vi "数据查询_仪器数据.vi"() -> ()   [LabVIEW 2016, in "数据查询.lvlib"]
uses:
  <vilib>/Utility/miscctls.llb/LVPointTypeDef.ctl
  <vilib>/Utility/miscctls.llb/LVRowAndColumnUnsignedTypeDef.ctl
  <userlib>/_OpenG.lib/array/array.llb/Sort 2D Array (String)__ogtk.vi
  <vilib>/ptbypt/NI_PtbyPt.lvlib
panel:
  in  "显示关键参数":bool
  in  "剔除异常数据":bool
  in  "数据类型":string(combo)="全部数据"
  in  "列表框":i32(listbox)
  in  "页":i32 format="第%.0f页"
  in  "每页条数":i32=1000
  in  "向后按钮":bool
  in  "向前按钮":bool
  in  "导出":bool
  in  "测量模式":string(combo)="全部数据"
  in  "查询":bool
  in  "结束日期":string="2050/01/01"
  in  "起始日期":string="2010/01/01"
  out "数据表":string[][](table)
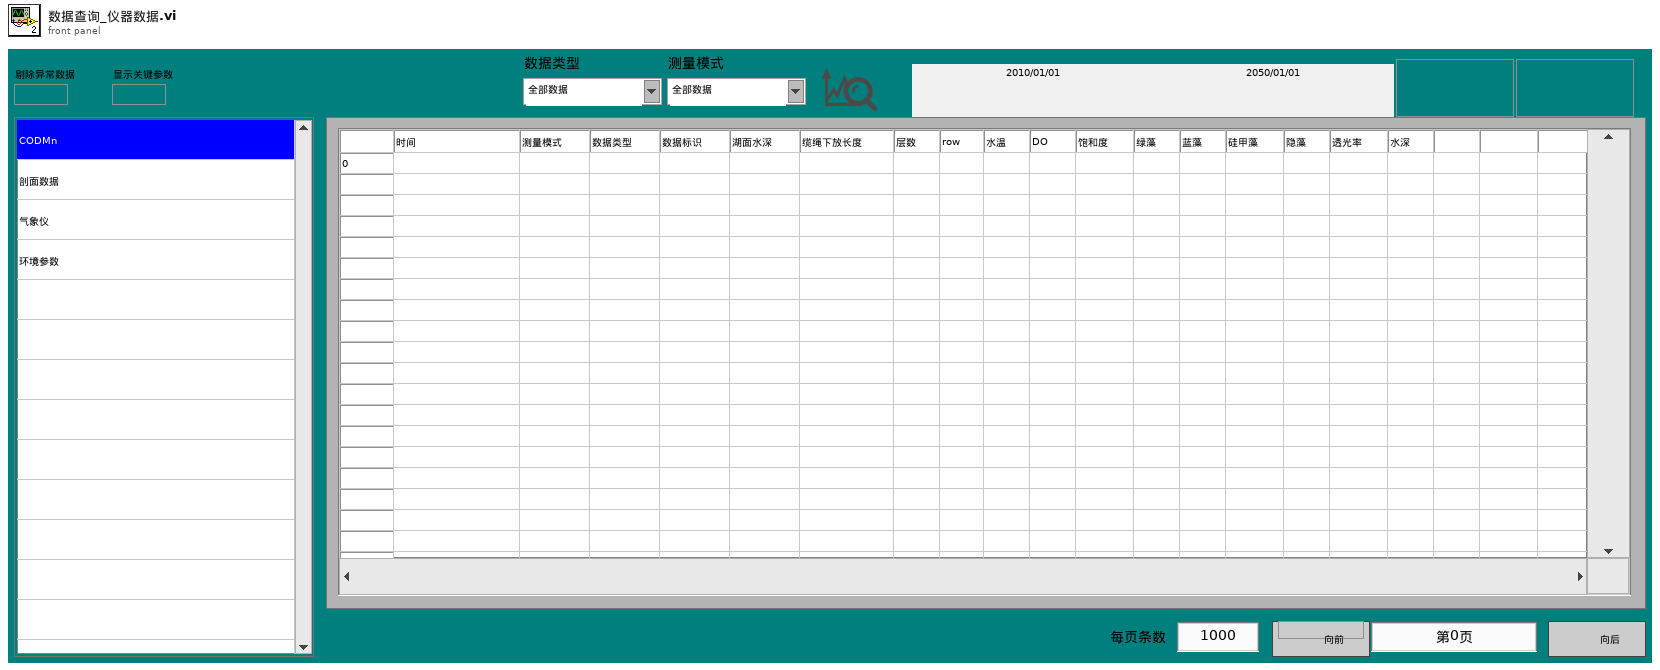
[diagram p1: front panel]
types:
  T1 = typedef "LVPointTypeDef.ctl" = cluster{"Horizontal":i16, "Vertical":i16}
  T2 = typedef "LVDateTimeRec.ctl" = cluster{"秒数的小数部分":dbl, "秒":i32, "分":i32, "时":i32, "日":i32, "月":i32, "年":i32, "天数（周）":i32, "天数（年）":i32, "DST":i32}
  T3 = typedef "数据查询菜单.xctl/数据 1.ctl" = enum32{"数据查询", "仪器数据", "仪器日志", "报警信息", "校准日志"}
  T4 = enum8{"Enabled", "Disabled", "Disabled and Grayed Out"}
  T5 = typedef "LVRowAndColumnUnsignedTypeDef.ctl" = cluster{"Row":u32, "Column":u32}
  T6 = typedef "数据库类型.ctl" = enum16{"Access", "SQLite"}
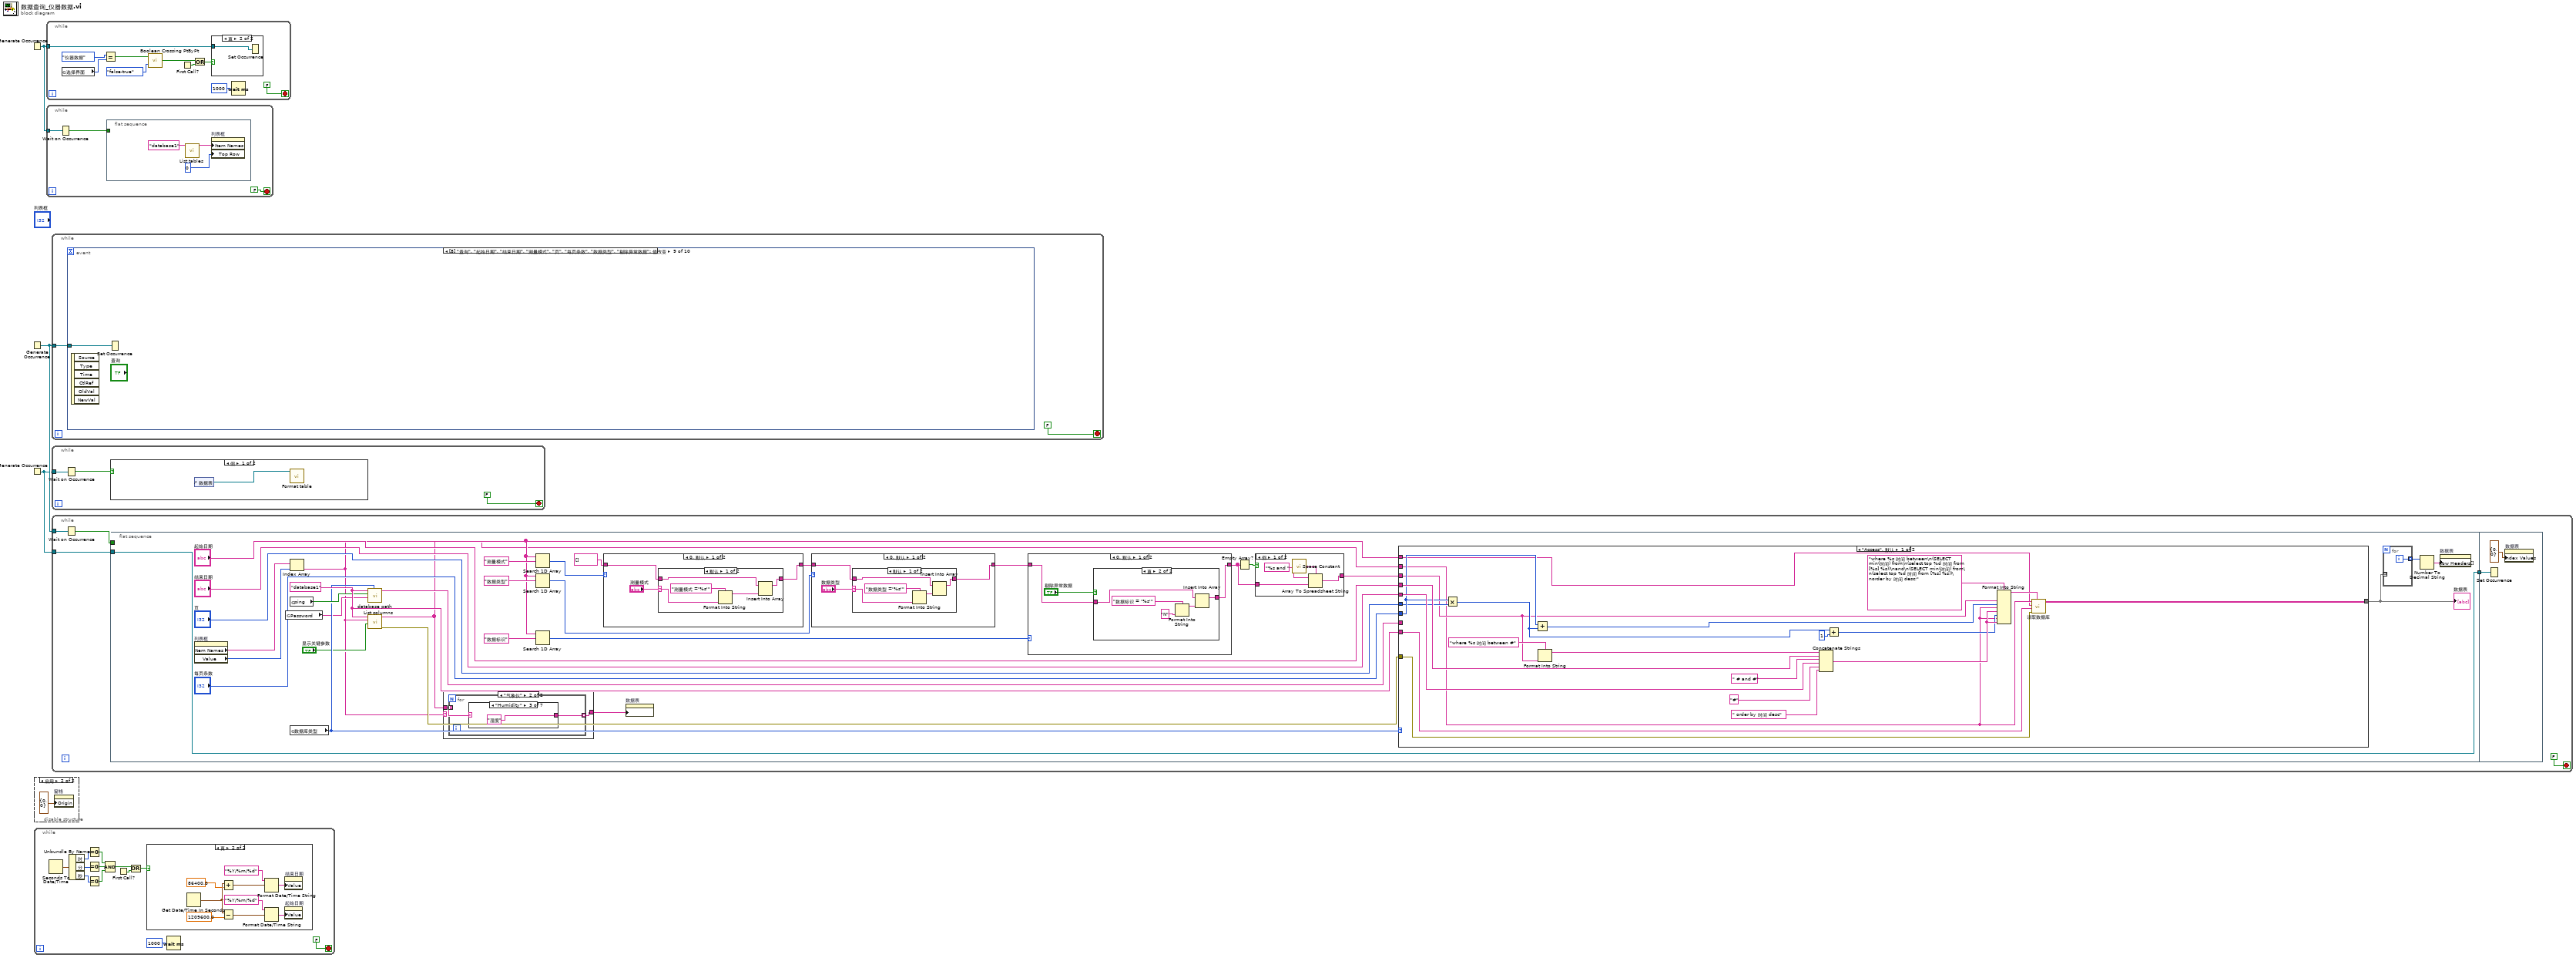
[diagram p0: block diagram]
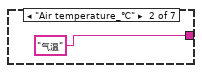
[diagram p6: hidden frame]
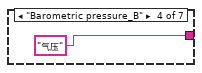
[diagram p7: hidden frame]
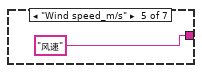
[diagram p8: hidden frame]
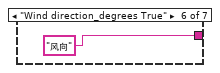
[diagram p9: hidden frame]
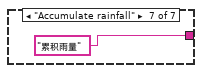
[diagram p10: hidden frame]
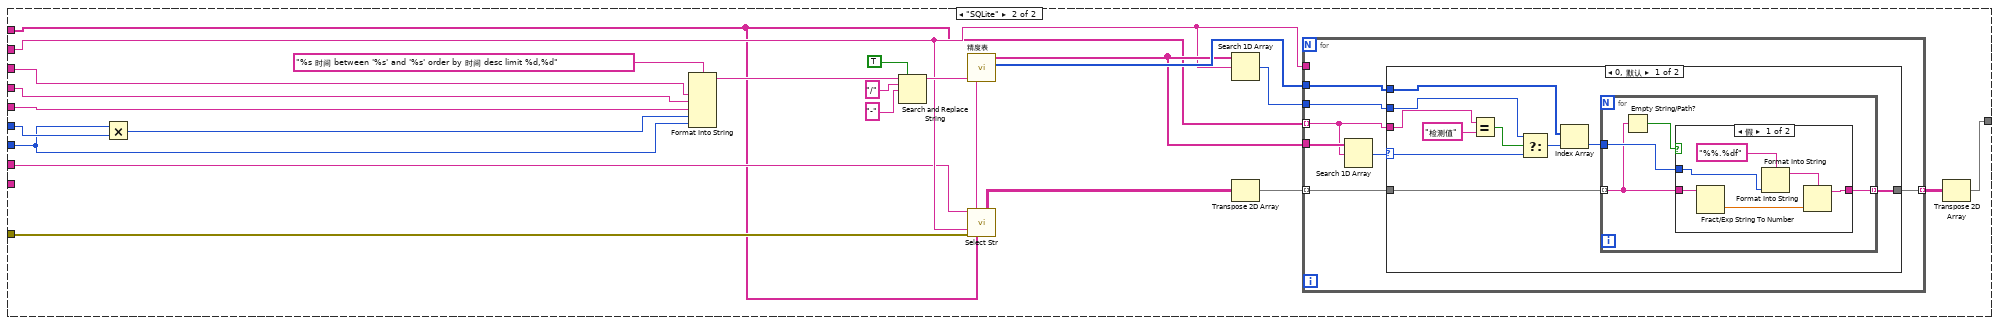
[diagram p11: hidden frame]
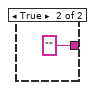
[diagram p14: hidden frame]
diagram:
  n1 = Generate Occurrence() -> (w1:refnum<k4>)
  n2 = Generate Occurrence() -> (w3:refnum<k4>)
  n3 = Generate Occurrence() -> (w2:refnum<k4>)
  n4 = disable-structure shown="启用" {
    frame Disabled {
    }
    frame Enabled {
      n5 = property on="窗格" class="Pane"("Origin"=T1 {"Horizontal"=0, "Vertical"=0} ("原点")) -> ()  [unwired: 2 in, 2 out]
    }
  }
  n6 = while {
    stop <- FALSE stop-if-true
    n7 = Seconds To Date/Time() -> (date time rec=w16:T2)  [unwired: 2 in]
    n8 = Unbundle By Name(w16) -> ("时"=w15:i32, "分"=w14:i32, "秒"=w13:i32)
    n9 = Equal To 0?(x=w15) -> (x = 0?=w12:bool)
    n10 = Equal To 0?(x=w14) -> (x = 0?=w11:bool)
    n11 = Equal To 0?(x=w13) -> (x = 0?=w10:bool)
    n12 = Compound Arithmetic op=AND ("复合运算")(w12, w11, w10) -> (w7:bool)
    n13 = First Call?() -> (First Call?: T/F=w6:bool)
    n14 = Or(x=w7, y=w6) -> (x .or. y?=w5:bool)
    n15 = case shown="真" w5 {
      frame False {
      }
      frame True {
        n16 = Get Date/Time In Seconds() -> (seconds since 1Jan1904=w21:timestamp)
        n17 = Add(x=w21, y=86400.0) -> (x+y=w19:timestamp)
        n18 = Subtract(x=w21, y=1209600.0) -> (x-y=w22:timestamp)
        n19 = Format Date/Time String(time format string (%c)="%Y/%m/%d" ("时间格式字符串(%c)"), seconds (now)=w19) -> (date/time string=w18:string)  [unwired: 1 in]
        n20 = Format Date/Time String(time format string (%c)="%Y/%m/%d" ("时间格式字符串(%c)"), seconds (now)=w22) -> (date/time string=w24:string)  [unwired: 1 in]
        n21 = property on="结束日期" class="Str"("Value"=w18) -> ()  [unwired: 2 in, 2 out]
        n22 = property on="起始日期" class="Str"("Value"=w24) -> ()  [unwired: 2 in, 2 out]
      }
    }
    n23 = Wait (ms)(milliseconds to wait=u32 1000 ("等待时间（毫秒）")) -> ()  [unwired: 1 out]
  }
  n24 = while {
    tunnel: w1 -> [w33]
    stop <- FALSE stop-if-true
    n25 = global read "全局变量.vi" "选择界面"() -> (w32:T3)
    n26 = Equal?(x=数据_1."仪器数据", y=w32) -> (x = y?=w30:bool)
    n27 = call <vilib>:"Boolean Crossing PtByPt.vi"("direction"=enum16{"either", "false-true", "true-false"}."false-true", "input"=w30) -> ("crossing"=w28:bool)  [unwired: 1 in]
    n28 = First Call?() -> (First Call?: T/F=w26:bool)
    n29 = Or(x=w28, y=w26) -> (x .or. y?=w27:bool)
    n30 = case shown="真" w27 {
      tunnel: w33 -> [_ w36]
      frame False {
      }
      frame True {
        n31 = Set Occurrence(w36) -> ()
      }
    }
    n32 = Wait (ms)(milliseconds to wait=u32 1000 ("等待时间（毫秒）")) -> ()  [unwired: 1 out]
  }
  n33 = while {
    tunnel: w1 -> [w38]
    stop <- FALSE stop-if-true
    n34 = Wait on Occurrence(2:w38) -> (0:w37:bool)  [unwired: 2 in]
    n35 = flat-sequence {
      tunnel: w37 -> [_]
      frame #0 {
        n36 = call "List tables.vi"("database"="database1") -> ("tables"=w40:string[])  [unwired: 9 in, 1 out]
        n37 = property on="列表框" class="LstBox (严格)"("Item Names"=w40, "Top Row"=0 ("顶行")) -> ()  [unwired: 2 in, 2 out]
      }
    }
  }
  n38 = while {
    tunnel: w3 -> [w43]
    stop <- FALSE stop-if-true
    n39 = event shown="[8] \"查询\", \"起始日期\", \"结束日期\", \"测量模式\", \"页\", \"每页条数\", \"数据类型\", \"剔除异常数据\": 值改变" {
      selector: _ -> [_ _ _ _ _ _ _ _ _ _]
      dyn-events: _ -> [_ _ _ _ _ _ _ _ _ _]
      timeout: _ -> [_ _ _ _ _ _ _ _ _ _]
      tunnel: w43 -> [_ _ _ _ _ _ _ _ w110 w112]
      event Timeout {
        n40 = event-data() -> ()  [unwired: 1 in, 3 out]
      }
      event "查询": Mouse Down {
        n41 = event-data() -> ()  [unwired: 1 in, 8 out]
        n42 = property on="页" class="DigNum (严格)"("Value"=0 ("页")) -> ()  [unwired: 2 in, 2 out]
      }
      event "每页条数": Mouse Down {
        n43 = event-data() -> ("CtlRef"=w47:refnum<vi>)  [unwired: 1 in, 7 out]
        n44 = property on="页" class="DigNum (严格)"("Value"=0 ("页")) -> ()  [unwired: 2 in, 2 out]
        n45 = property class="DigNum (严格)"(reference=w47) -> (reference out=w48:refnum<vi>, "Value"=w50:i32)  [unwired: 1 in, 1 out]
        n46 = call "数字键盘.vi"("OldNumber"=w50) -> ("NewNumber"=w49:sgl)
        n47 = property class="DigNum (严格)"(reference=w48, "Val(Sgnl)"=w49) -> ()  [unwired: 1 in, 2 out]
      }
      event "页": Mouse Down {
        n48 = event-data() -> ("CtlRef"=w51:refnum<vi>)  [unwired: 1 in, 7 out]
        n49 = property class="DigNum (严格)"(reference=w51) -> (reference out=w52:refnum<vi>, "Value"=w54:i32)  [unwired: 1 in, 1 out]
        n50 = call "数字键盘.vi"("OldNumber"=w54) -> ("NewNumber"=w53:sgl)
        n51 = property class="DigNum (严格)"(reference=w52, "Val(Sgnl)"=w53) -> ()  [unwired: 1 in, 2 out]
      }
      event "向前按钮": Value Change {
        n52 = event-data() -> ()  [unwired: 1 in, 6 out]
        n53 = property on="页" class="DigNum (严格)"() -> ("Value"=w60:i32)  [unwired: 2 in, 2 out]
        n54 = Decrement(x=w60) -> (x-1=w59:i32)
        n55 = In Range and Coerce(upper limit=9999 ("上限"), x=w59, lower limit=0 ("下限")) -> (coerced(x)=w56:i32, In Range?=w55:bool)
        n56 = case shown="真" w55 {
          tunnel: w56 -> [_ w61]
          frame False {
          }
          frame True {
            n57 = property on="页" class="DigNum (严格)"("Val(Sgnl)"=w61) -> ()  [unwired: 2 in, 2 out]
          }
        }
      }
      event "向后按钮": Value Change {
        n58 = event-data() -> ()  [unwired: 1 in, 6 out]
        n59 = property on="页" class="DigNum (严格)"() -> ("Value"=w66:i32)  [unwired: 2 in, 2 out]
        n60 = Increment(x=w66) -> (x+1=w65:i32)
        n61 = In Range and Coerce(upper limit=u32 9999 ("上限"), x=w65, lower limit=u32 0 ("下限")) -> (coerced(x)=w62:u32)  [unwired: 1 out]
        n62 = property on="页" class="DigNum (严格)"("Val(Sgnl)"=w62) -> ()  [unwired: 2 in, 2 out]
      }
      event "导出": Value Change {
        n63 = event-data() -> ("CtlRef"=w67:refnum<vi>)  [unwired: 1 in, 5 out]
        n64 = property class="Bool"(reference=w67, "DisabledEnum"=T4."Disabled and Grayed Out" ("禁用")) -> (reference out=w71:refnum<vi>, error out=w72:errorcluster)  [unwired: 1 in]
        n65 = flat-sequence {
          tunnel: w72 -> [_]
          tunnel: [w91] -> w70
          tunnel: w71 -> [w91]
          tunnel: "导出" -> [_]
          frame #0 {
            n66 = property on="列表框" class="LstBox (严格)"() -> ("Item Names"=w76:string[], "Value"=w75:i32)  [unwired: 2 in, 2 out]
            n67 = local read "数据表"() -> (w95:string[][])
            n68 = Index Array(array=w76, index=w75) -> (element=w74:string)
            n69 = Format Date/Time String(time format string (%c)="%y_%m_%d" ("时间格式字符串(%c)")) -> (date/time string=w88:string)  [unwired: 2 in]
            n70 = call-poly <userlib>:"Sort Array__ogtk.vi"("Column/Row to Sort By"=u32 0, "Sort By in"=enum16{"row", "column"}."column", "Order"=enum16{"ascending", "descending"}."ascending", "Array in"=w95) -> ("Sorted Array out"=w77:string[][])  [unwired: 4 in, 3 out]
            n71 = Concatenate Strings(w74, "_" ("字符串"), w88) -> (w86:string)
            n72 = for {
              tunnel: w77 -> [w104] mode=indexing
              tunnel: [w103] -> w81 mode=indexing
              i -> [w105]
              n73 = Increment(x=w105) -> (x+1=w101:i32)
              n74 = Number To Decimal String(number=w101) -> (decimal integer string=w100:string)  [unwired: 1 in]
              n75 = Insert Into Array(array=w104, index=0 ("索引"), new element=w100) -> (w103:string[])
            }
            n76 = property on="数据表" class="Tbl (严格)"() -> ("Column Headers[]"=w84:string[])  [unwired: 2 in, 2 out]
            n77 = Insert Into Array(array=w84, index=0 ("索引"), new element="序号" ("新元素/子数组")) -> (w85:string[])
            n78 = Insert Into Array(array=string[][] [], new element #1=w85, new element #2=w81) -> (w80:string[][])  [unwired: 2 in]
            n79 = call "数据导出Excel.vi"("text data"=w80, "default name"=w86) -> ("error out"=w79:errorcluster, "布尔"=w78:bool)  [unwired: 8 in]
            n80 = case shown="真" w78 {
              tunnel: w79 -> [_ w97]
              frame False {
              }
              frame True {
                n81 = case shown="错误" w97 {
                  tunnel: ["导出成功" ("消息") "导出失败" ("消息")] -> w96
                  frame No Error {
                  }
                  frame Error {
                  }
                }
                n82 = One Button Dialog(message=w96) -> ()  [unwired: 1 in, 1 out]
              }
            }
          }
        }
        n83 = property class="Bool"(reference=w70, "DisabledEnum"=T4."Enabled" ("禁用")) -> ()  [unwired: 1 in, 2 out]
      }
      event "起始日期", "结束日期": Mouse Down {
        n84 = event-data() -> ("CtlRef"=w109:refnum<vi>)  [unwired: 1 in, 7 out]
        n85 = property class="Str"(reference=w109) -> (reference out=w107:refnum<vi>, "Value"=w108:string)  [unwired: 1 in, 1 out]
        n86 = call "日期键盘.vi"("原值"=w108) -> ("x+y"=w106:string)  [unwired: 10 in]
        n87 = property class="Str"(reference=w107, "Val(Sgnl)"=w106) -> ()  [unwired: 1 in, 2 out]
      }
      event "查询", "起始日期", "结束日期", "测量模式", "页", "每页条数", "数据类型", "剔除异常数据": Value Change {
        n88 = event-data() -> ()  [unwired: 1 in, 6 out]
        n89 = Set Occurrence(w110) -> ()
      }
      event "列表框": Value Change; "列表框": Mouse Down {
        n90 = event-data() -> ()  [unwired: 1 in, 4 out]
        n91 = flat-sequence {
          tunnel: w112 -> [w115]
          tunnel: [w115] -> w111
          tunnel: w111 -> [w116]
          frame #0 {
            n92 = property on="测量模式" class="CmbBox"("Value"="全部数据" ("测量模式")) -> ()  [unwired: 2 in, 2 out]
            n93 = property on="数据类型" class="CmbBox"("Value"="全部数据" ("数据类型")) -> ()  [unwired: 2 in, 2 out]
          }
          frame #1 {
            n94 = Set Occurrence(w116) -> ()
          }
        }
      }
    }
  }
  n95 = while {
    tunnel: w2 -> [w117]
    stop <- FALSE stop-if-true
    n96 = Wait on Occurrence(2:w117) -> (0:w119:bool)  [unwired: 2 in]
    n97 = case shown="假" w119 {
      frame False {
        n98 = control-ref of="数据表"() -> (w120:refnum<vi>)
        n99 = call "Format table.vi"("Table输入"=w120) -> ()  [unwired: 11 in]
      }
      frame True {
      }
    }
  }
  n100 = while {
    tunnel: w3 -> [w124]
    tunnel: w2 -> [w121]
    stop <- FALSE stop-if-true
    n101 = Wait on Occurrence(2:w124) -> (0:w123:bool)  [unwired: 2 in]
    n102 = flat-sequence {
      tunnel: w123 -> [_]
      tunnel: w121 -> [w146]
      tunnel: [w146] -> w122
      tunnel: w122 -> [w280]
      frame #0 {
        w134 = "database1" ("database")
        n103 = property on="列表框" class="LstBox (严格)"() -> ("Item Names"=w145:string[], "Value"=w151:i32)  [unwired: 2 in, 2 out]
        n104 = global read "全局变量.vi" "Password"() -> (w129:string)
        n105 = Index Array(array=w145, index=w151) -> (element=w127:string)
        n106 = global read "全局变量.vi" "ping"() -> (w132:bool)
        n107 = global read "全局变量.vi" "数据库类型"() -> (w131:T6)
        n108 = call "database path.vi"("数据库类型"=w131, "Password"=w129, "ping"=w132, "database"=w134) -> ("Path out"=w133:string)  [unwired: 6 in, 1 out]
        n109 = call "List columns.vi"("显示关键参数"="显示关键参数", "table"=w127, "database"=w134) -> ("error out"=w144:errorcluster, "columns"=w128:string[])  [unwired: 7 in]
        n110 = case shown="\"气象仪\"" w127 {
          tunnel: w128 -> [w158 w160]
          tunnel: [w158 w159] -> w126
          frame "假", Default {
          }
          frame "气象仪" {
            n111 = for {
              tunnel: w160 -> [w162] mode=indexing
              tunnel: [w161] -> w159 mode=indexing
              n112 = case shown="\"Humidity\"" w162 {
                selector: w162 -> [w163 _ _ _ _ _ _]
                tunnel: [w163 "气温" "湿度" "气压" "风速" "风向" "累积雨量"] -> w161
                frame "", Default {
                }
                frame "Air temperature_℃" {
                }
                frame "Humidity" {
                }
                frame "Barometric pressure_B" {
                }
                frame "Wind speed_m/s" {
                }
                frame "Wind direction_degrees True" {
                }
                frame "Accumulate rainfall" {
                }
              }
            }
          }
        }
        n113 = Search 1D Array(1D array=w128, element="测量模式" ("元素")) -> (index of element=w138:i32)  [unwired: 1 in]
        n114 = Search 1D Array(1D array=w128, element="数据类型" ("元素")) -> (index of element=w141:i32)  [unwired: 1 in]
        n115 = Search 1D Array(1D array=w128, element="数据标识" ("元素")) -> (index of element=w139:i32)  [unwired: 1 in]
        n116 = case shown="0, 默认" w138 {
          tunnel: string[] [] -> [w251 w258]
          tunnel: [w249 w258] -> w148
          frame 0, Default {
            n117 = case shown="默认" "测量模式" {
              selector: "测量模式" -> [w252 _]
              tunnel: w251 -> [w255 w257]
              tunnel: [w253 w257] -> w249
              frame Default {
                n118 = Format Into String(format string="测量模式 ='%s'" ("condition"), w252) -> (resulting string=w254:string)  [unwired: 2 in, 1 out]
                n119 = Insert Into Array(array=w255, new element=w254) -> (w253:string[])  [unwired: 1 in]
              }
              frame "全部数据" {
              }
            }
          }
          frame -1 {
          }
        }
        n120 = property on="数据表" class="Tbl (严格)"("Column Headers[]"=w126) -> ()  [unwired: 2 in, 2 out]
        n121 = case shown="0, 默认" w141 {
          tunnel: w148 -> [w271 w278]
          tunnel: [w270 w278] -> w143
          frame 0, Default {
            n122 = case shown="默认" "数据类型" {
              selector: "数据类型" -> [w272 _]
              tunnel: w271 -> [w275 w277]
              tunnel: [w273 w277] -> w270
              frame Default {
                n123 = Format Into String(format string="数据类型 ='%s'" ("condition"), w272) -> (resulting string=w274:string)  [unwired: 2 in, 1 out]
                n124 = Insert Into Array(array=w275, new element=w274) -> (w273:string[])  [unwired: 1 in]
              }
              frame "全部数据" {
              }
            }
          }
          frame -1 {
          }
        }
        n125 = case shown="0, 默认" w139 {
          tunnel: [w261 w268] -> w136
          tunnel: w143 -> [w259 w268]
          frame 0, Default {
            n126 = case shown="真" "剔除异常数据" {
              tunnel: w259 -> [w262 w267]
              tunnel: [w262 w266] -> w261
              frame False {
              }
              frame True {
                n127 = Format Into String(format string="数据标识 = '%s'" ("condition"), "N" ("String")) -> (resulting string=w263:string)  [unwired: 2 in, 1 out]
                n128 = Insert Into Array(array=w267, new element=w263) -> (w266:string[])  [unwired: 1 in]
              }
            }
          }
          frame -1 {
          }
        }
        n129 = Empty Array?(array=w136) -> (empty?=w135:bool)
        n130 = case shown="假" w135 {
          tunnel: [w245 "" ("spreadsheet string")] -> w147
          tunnel: w136 -> [w244 _]
          frame False {
            n131 = call <vilib>:"Space Constant.vi"() -> ("String"=w247:string)
            n132 = Array To Spreadsheet String(delimiter (Tab)=w247, array=w244, 3:"%s and " ("格式字符串")) -> (spreadsheet string=w245:string)
          }
          frame True {
          }
        }
        n133 = case shown="\"Access\", 默认" w131 {
          tunnel: "起始日期" -> [w191 w211]
          tunnel: "结束日期" -> [w190 w210]
          tunnel: "每页条数" -> [w183 w208]
          tunnel: "页" -> [w182 w209]
          tunnel: [w181 w198] -> w150
          tunnel: w147 -> [w174 w212]
          tunnel: w144 -> [w173 w214]
          tunnel: w127 -> [w172 w195]
          tunnel: w134 -> [w171 _]
          tunnel: w128 -> [w170 w192]
          tunnel: w133 -> [_ w193]
          frame "Access", Default {
            n134 = Multiply(x=w183, y=w182) -> (x*y=w179:i32)
            n135 = Add(x=w183, y=w179) -> (x+y=w177:i32)
            n136 = Format Into String(format string="where %s 时间 between #" ("condition"), w174) -> (resulting string=w187:string)  [unwired: 2 in, 1 out]
            n137 = Concatenate Strings(w187, w191, " # and #" ("condition"), w190, "#" ("condition"), " order by 时间 desc" ("字符串")) -> (w185:string)
            n138 = Add(x=w179, y=u32 1) -> (x+y=w176:u32)
            n139 = Format Into String(format string="where %s 时间 between\n(SELECT min(时间) from\n(select top %d 时间 from [%s] %s))\nand\n(SELECT min(时间) from\n(select top %d 时间 from [%s] %s))\norder by 时间 desc;" ("格式字符串"), w174, w177, w172, w185, w176, w172, w185) -> (resulting string=w184:string)  [unwired: 2 in, 1 out]
            n140 = call "读取数据库.vi"("condition"=w184, "error in (no error)"=w173, "database"=w171, "显示项"=w170, "组合框"=w172) -> ("表格"=w181:string[][])  [unwired: 3 in, 3 out]
          }
          frame "SQLite" {
            n141 = Multiply(x=w208, y=w209) -> (x*y=w207:i32)
            n142 = Format Into String(format string="%s 时间 between '%s' and '%s' order by 时间 desc limit %d,%d" ("格式字符串"), w212, w211, w210, w207, w208) -> (resulting string=w203:string)  [unwired: 2 in, 1 out]
            n143 = Search and Replace String(replace all?=TRUE ("替换全部？(F)"), input string=w203, search string="/" ("搜索字符串"), replace string="-" ("替换字符串(\"\")")) -> (result string=w202:string)  [unwired: 4 in, 3 out]
            n144 = call "精度表.vi"() -> ("精度"=w197:i32[], "参数"=w196:string[])  [unwired: 10 in]
            n145 = call "Select Str.vi"("DB Path"=w193, "Where Clause"=w202, "Tables Name"=w195, "error in (no error)"=w214, "Columns"=w192) -> ("Results"=w201:string[][])  [unwired: 7 in, 3 out]
            n146 = Search 1D Array(1D array=w196, element=w195) -> (index of element=w194:i32)  [unwired: 1 in]
            n147 = Transpose 2D Array(2D array=w201) -> (transposed array=w200:string[][])
            n148 = for {
              tunnel: w192 -> [w216] mode=indexing
              tunnel: w200 -> [w221] mode=indexing
              tunnel: [w220] -> w199 mode=indexing
              tunnel: w195 -> [_]
              tunnel: w196 -> [w217]
              tunnel: w197 -> [w219]
              tunnel: w194 -> [w215]
              n149 = Search 1D Array(1D array=w217, element=w216) -> (index of element=w218:i32)  [unwired: 1 in]
              n150 = case shown="0, 默认" w218 {
                selector: w218 -> [w223 _]
                tunnel: w221 -> [w231 w243]
                tunnel: [w230 w243] -> w220
                tunnel: w219 -> [w229 _]
                tunnel: w216 -> [w226 _]
                tunnel: w215 -> [w224 _]
                frame 0, Default {
                  n151 = Equal?(x=w226, y="检测值" ("元素")) -> (x = y?=w225:bool)
                  n152 = Select(t=w224, s=w225, f=w223) -> (s? t:f=w222:i32)
                  n153 = Index Array(array=w229, index=w222) -> (element=w228:i32)
                  n154 = for {
                    tunnel: w231 -> [w233] mode=indexing
                    tunnel: [w234] -> w230 mode=indexing
                    tunnel: w228 -> [w235]
                    n155 = Empty String/Path?(string/path=w233) -> (empty?=w232:bool)
                    n156 = case shown="假" w232 {
                      tunnel: w235 -> [w240 _]
                      tunnel: [w237 w242] -> w234
                      tunnel: w233 -> [w236 w242]
                      frame False {
                        n157 = Fract/Exp String To Number(string=w236) -> (number=w241:dbl)  [unwired: 3 in, 1 out]
                        n158 = Format Into String(format string="%%.%df" ("格式字符串"), w240) -> (resulting string=w239:string)  [unwired: 2 in, 1 out]
                        n159 = Format Into String(format string=w239, w241) -> (resulting string=w237:string)  [unwired: 2 in, 1 out]
                      }
                      frame True {
                      }
                    }
                  }
                }
                frame -1 {
                }
              }
            }
            n160 = Transpose 2D Array(2D array=w199) -> (transposed array=w198:string[][])
          }
        }
        "数据表" <- w150
        n161 = for {
          tunnel: w150 -> [_] mode=indexing
          tunnel: [w279] -> w155 mode=indexing
          i -> [w279]
        }
        n162 = Number To Decimal String(number=w155) -> (decimal integer string=w154:string[])  [unwired: 1 in]
        n163 = property on="数据表" class="Tbl (严格)"("Row Headers[]"=w154) -> ()  [unwired: 2 in, 2 out]
      }
      frame #1 {
        n164 = Set Occurrence(w280) -> ()
        n165 = property on="数据表" class="Tbl (严格)"("Index Values"=T5 {"Row"=0, "Column"=0} ("索引值")) -> ()  [unwired: 2 in, 2 out]
      }
    }
  }
